vi "Check Sampling Rate and Record Length Support.vi"(0 "Scope Reference":refnum<k15>, 1 "Autoset Sampling Rate?":bool=TRUE, 5 "Frequency Sweep":dbl format="%#_6p", 7 "Resolution Bandwidth(%)":dbl min=0.0 max=100.0, 9 "Sampling Rate Multiplier":dbl=2.0 min=2.0 max=100.0, 11 "error in":errorcluster) -> (4 "Scope Reference Out":refnum<k15>, 6 "Minimum Sampling Rate":dbl, 8 "Minimum Record Length":i32, 10 "Parameter Supported?":bool=TRUE, 13 "Maximum Record length":i32, 14 "Maximum Sampling Rate":dbl, 15 "error out":errorcluster)   [LabVIEW 2020, in "LDO PSRR.lvlib"]
uses:
  LDO PSRR.lvlib
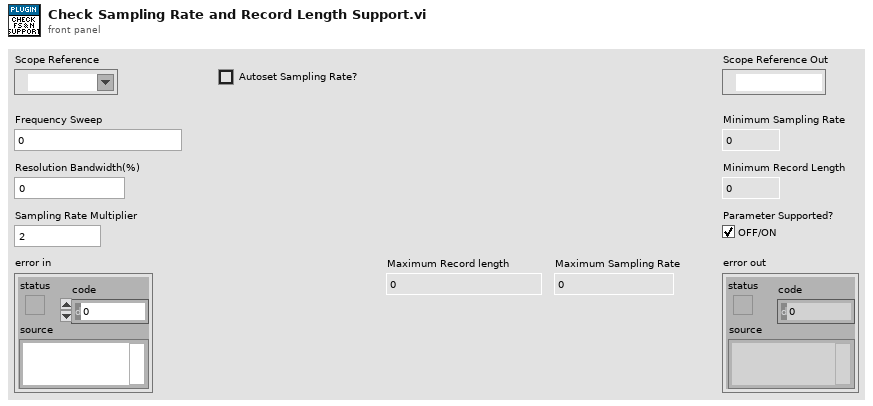
[diagram p1: front panel]
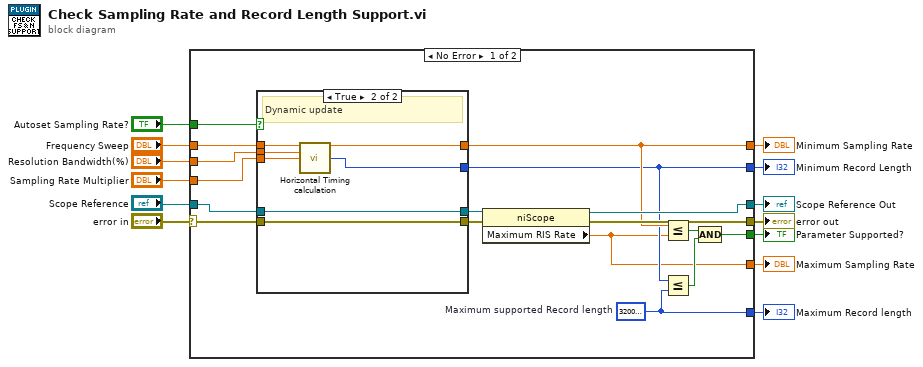
[diagram p0: block diagram]
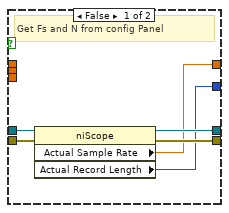
[diagram p2: hidden frame]
diagram:
  n1 = case shown="No Error" "error in" {
    selector: "error in" -> [w16 w45]
    tunnel: "Frequency Sweep" -> [w30 _]
    tunnel: "Resolution Bandwidth(%)" -> [w29 _]
    tunnel: "Sampling Rate Multiplier" -> [w28 _]
    tunnel: [w25 w45] -> w9
    tunnel: "Scope Reference" -> [w18 w44]
    tunnel: [w24 w44] -> w7
    tunnel: [w23 _] -> w6
    tunnel: [w22 _] -> w5
    tunnel: [w21 _] -> w4
    tunnel: [w20 _] -> w2
    tunnel: "Autoset Sampling Rate?" -> [w15 _]
    tunnel: [w14 _] -> w1
    frame No Error {
      w14 = 32000000  # Maximum supported Record length
      n2 = case shown="True" w15 {
        tunnel: w30 -> [_ w43]
        tunnel: w29 -> [_ w42]
        tunnel: w28 -> [_ w41]
        tunnel: [w32 w40] -> w23
        tunnel: [w31 w39] -> w22
        tunnel: [w33 w37] -> w19
        tunnel: w18 -> [w34 w37]
        tunnel: [w35 w38] -> w17
        tunnel: w16 -> [w36 w38]
        frame False {
          # "Get Fs and N from config Panel"
          n3 = property class="niScope"(reference=w34, error in=w36) -> (reference out=w33:refnum<k15>, error out=w35:errorcluster, "Actual Sample Rate"=w32:dbl, "Actual Record Length"=w31:i32)
        }
        frame True {
          # "Dynamic update"
          n4 = call "Horizontal Timing calculation.vi"("Frequency Sweep"=w43, "Resolution Bandwidth(%)"=w42, "Sampling Rate Multiplier"=w41) -> ("Minimum Sampling Rate"=w40:dbl, "Minimum Record Length"=w39:i32)  [unwired: 11 in]
        }
      }
      n5 = property class="niScope"(reference=w19, error in=w17) -> (reference out=w24:refnum<k15>, error out=w25:errorcluster, "Maximum RIS Rate"=w20:dbl)
      n6 = Less Or Equal?(x=w23, y=w20) -> (x <= y?=w27:bool)
      n7 = Less Or Equal?(x=w22, y=w14) -> (x <= y?=w26:bool)
      n8 = Compound Arithmetic op=AND(w27, w26) -> (w21:bool)
    }
    frame Error {
    }
  }
  "error out" <- w9
  "Scope Reference Out" <- w7
  "Parameter Supported?" <- w4
  "Minimum Sampling Rate" <- w6
  "Minimum Record Length" <- w5
  "Maximum Sampling Rate" <- w2
  "Maximum Record length" <- w1
